vi "Copy.vi"(11 "TypedCircularBuffer in":refnum<class "VarCircularBuffer.lvclass">) -> (2 "Copied Buffer":variant[](array[variant]), 3 "TypedCircularBuffer out":refnum<class "VarCircularBuffer.lvclass">)   [LabVIEW 2024, in "VarCircularBuffer.lvclass"]
uses:
  VarCircularBuffer.lvclass
  VarCircularBuffer.lvclass/VarCircularBuffer.ctl
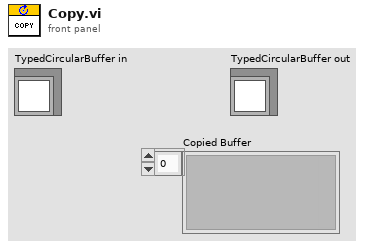
[diagram p1: front panel]
types:
  T1 = typedef "VarCircularBuffer.lvclass/Type.ctl" = variant
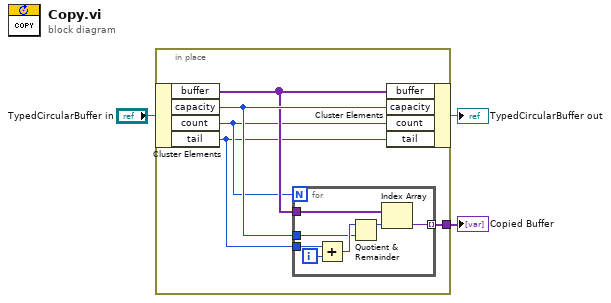
[diagram p0: block diagram]
diagram:
  n1 = in-place {
    in-place-border: [w8] -> w1
    n2 = in-place-cluster #1("TypedCircularBuffer in") -> ("buffer"=w6:T1[], "capacity"=w7:u32, "count"=w5:u32, "tail"=w4:u32)
    n3 = for {
      N: w5 -> [_]
      tunnel: w6 -> [w15]
      tunnel: w4 -> [w13]
      tunnel: w7 -> [w10]
      tunnel: [w9] -> w8 mode=indexing
      i -> [w14]
      n4 = Add(x=w13, y=w14) -> (x+y=w12:u32)
      n5 = Quotient & Remainder(x=w12, y=w10) -> (x-y*floor(x/y)=w11:u32)  [unwired: 1 out]
      n6 = Index Array(array=w15, index=w11) -> (element=w9:T1)
    }
    n7 = in-place-cluster #1("buffer"=w6, "capacity"=w7, "count"=w5, "tail"=w4) -> (→"TypedCircularBuffer out":refnum<class "VarCircularBuffer.lvclass">)
  }
  "Copied Buffer" <- w1
